vi "XML_FF_writeTrial.vi"(8 "error in (no error)":errorcluster, 9 "Trial Number":i32, 10 "XML_FF_Trial":T1, 11 "DOM document in":refnum<k20>) -> (0 "error out":errorcluster, 3 "DOM document out":refnum<k20>)   [LabVIEW 2016, in "XML_EEG_Features.lvlib"]
uses:
  XML_EEG_Features.lvlib
  XML_FF_Trial.ctl
  <vilib>/xml/NI_XML.lvlib
  <resource>/objmgr/DOMUserDefRef.rc
panel:
  # "This VI is a part of BCI Design library, http://www.ru-bci.org \nCopyright © 2020, Sotnikov Peter, All rights reserved. License: CC BY-NC 4.0"
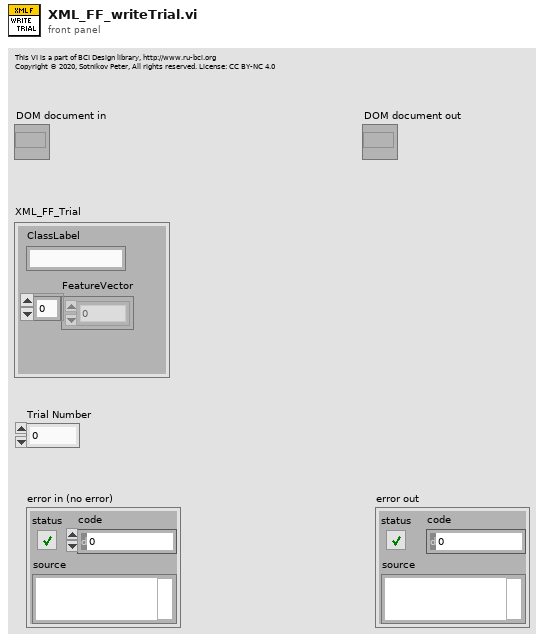
[diagram p1: front panel]
types:
  T1 = typedef "XML_EEG_Features.lvlib/XML_FF_Trial.ctl" = cluster{"ClassLabel":string, "FeatureVector":dbl[]}
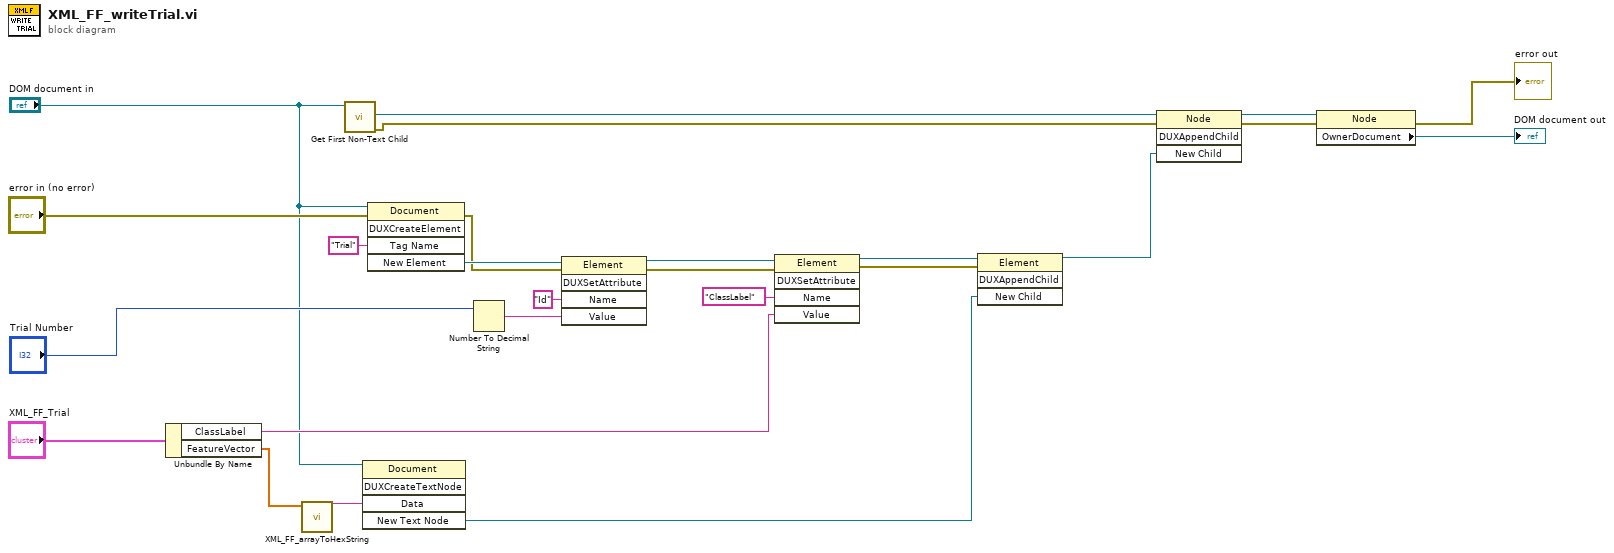
[diagram p0: block diagram]
diagram:
  n1 = Unbundle By Name("XML_FF_Trial") -> ("ClassLabel"=w16:string, "FeatureVector"=w13:dbl[])
  n2 = call "XML_FF_arrayToHexString.vi"("Array"=w13) -> ("HexString out"=w12:string)  [unwired: 9 in, 1 out]
  n3 = call <vilib>:"Get First Non-Text Child.vi"("node in"="DOM document in") -> ("error out"=w4:errorcluster, "child node"=w7:refnum<k20>)  [unwired: 7 in, 2 out]
  n4 = invoke class="Document" method="DUXCreateTextNode"(reference="DOM document in", "Data"=w12) -> ("New Text Node"=w9:refnum<k20>)  [unwired: 3 in, 4 out]
  n5 = invoke class="Document" method="DUXCreateElement"(reference="DOM document in", error in="error in (no error)", "Tag Name"="Trial") -> (error out=w15:errorcluster, "New Element"=w22:refnum<k20>)  [unwired: 2 in, 3 out]
  n6 = Number To Decimal String(number="Trial Number") -> (decimal integer string=w20:string)  [unwired: 1 in]
  n7 = invoke class="Element" method="DUXSetAttribute"(reference=w22, error in=w15, "Name"="Id", "Value"=w20) -> (reference out=w18:refnum<k20>, error out=w14:errorcluster)  [unwired: 1 in, 3 out]
  n8 = invoke class="Element" method="DUXSetAttribute"(reference=w18, error in=w14, "Name"="ClassLabel", "Value"=w16) -> (reference out=w10:refnum<k20>, error out=w8:errorcluster)  [unwired: 1 in, 3 out]
  n9 = invoke class="Element" method="DUXAppendChild"(reference=w10, error in=w8, "New Child"=w9) -> (reference out=w6:refnum<k20>)  [unwired: 1 in, 3 out]
  n10 = invoke class="Node" method="DUXAppendChild"(reference=w7, error in=w4, "New Child"=w6) -> (reference out=w5:refnum<k20>, error out=w3:errorcluster)  [unwired: 1 in, 2 out]
  n11 = property class="Node"(reference=w5, error in=w3) -> (error out=→"error out":errorcluster, "OwnerDocument"=→"DOM document out":refnum<k20>)  [unwired: 1 out]
